vi "Process.vi"(8 "error in":errorcluster, 11 "Plugin in":refnum<class "Tone Measurements.lvclass">) -> (0 "error out":errorcluster, 3 "Plugin out":refnum<class "Tone Measurements.lvclass">)   [LabVIEW 2025, in "Tone Measurements.lvlib" / "Tone Measurements.lvclass"]
uses:
  Tone Measurements.lvclass
  C:/Program Files/National Instruments/LabVIEW 2025/vi.lib/FlexLogger/SDK/PluginSDK.lvlibp/PEFClasses/SDK/Plugin/Plugin.lvclass
  <vilib>/addons/_NISVFA/_Shared subVIs/Controls/svc_Window.ctl
  Tone Measurements.lvclass/Tone Measurements.ctl
  <vilib>/addons/_NISVFA/_Shared subVIs/Data Objects/Data/Data.lvclass/Data.ctl
  <vilib>/addons/_NISVFA/_Shared subVIs/Data Objects/Data/Read Data Increment.vi
  <vilib>/addons/_NISVFA/_Shared subVIs/Data Objects/Data/Read Data Attributes.vi
  <vilib>/addons/_NISVFA/_Shared subVIs/Data Objects/subVIs/Get Data Sample Interval (dt).vi
  <vilib>/addons/_NISVFA/_Shared subVIs/Common/sv_Get NI Property Name String.vi
  <vilib>/addons/_NISVFA/_Shared subVIs/Data Objects/Waveforms (DBL)/Waveforms (N Ch).lvclass
  C:/Program Files/NI/LVAddons/nisvt/1/vi.lib/addons/_NISVFA/_Shared subVIs/Data Objects/Data/Data.lvclass
  <vilib>/addons/_NISVFA/_Shared subVIs/Data Objects/Waveforms (DBL)/SV Read Newest Data.vi
  <vilib>/FlexLogger/SDK/PluginSDK.lvlibp/PEFClasses/SDK/Plugin/DataHelpers/Write 1D Wfm (DBL)_v2.vi
  C:/Program Files/National Instruments/LabVIEW 2025/vi.lib/FlexLogger/SDK/PluginSDK.lvlibp/PEFClasses/SDK/Processing Element/Processing Element.lvclass
  C:/dev/dsb/niflexlogger-plugins/PDK plugins/Tone Measurements/Tone Measurements.lvclass
  <vilib>/FlexLogger/SDK/PluginSDK.lvlibp/PEFClasses/SDK/Plugin/Plugin.lvclass
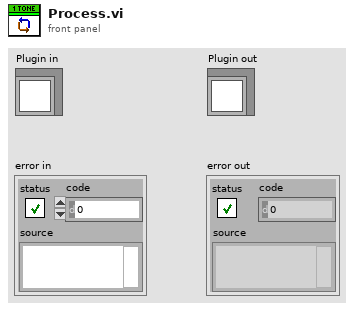
[diagram p1: front panel]
types:
  T1 = cluster{"start frequency":dbl, "stop frequency":dbl}
  T2 = typedef "svc_Window.ctl" = u32
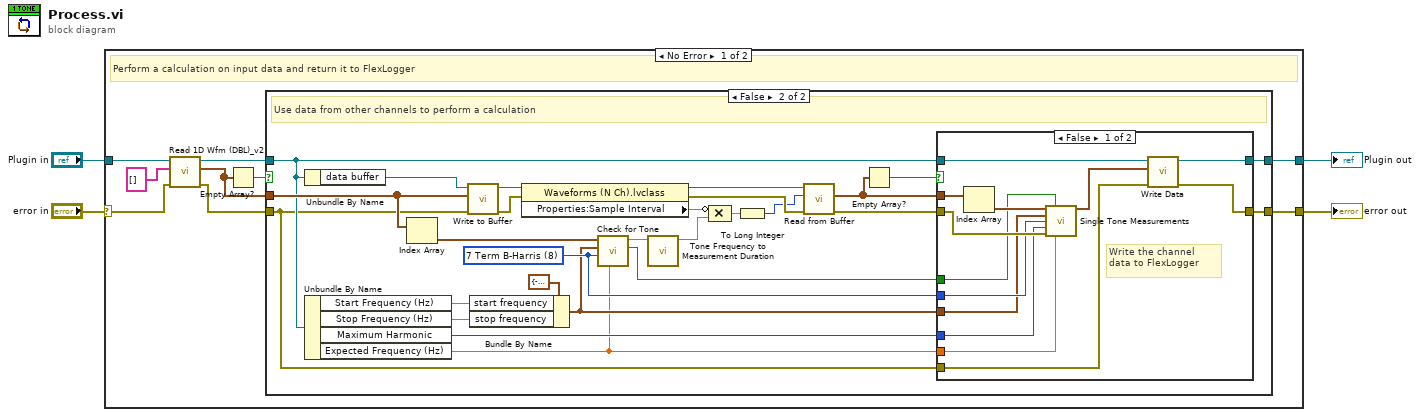
[diagram p0: block diagram]
diagram:
  n1 = case shown="No Error" "error in" {
    selector: "error in" -> [w12 w58]
    tunnel: [w10 w59] -> w1
    tunnel: "Plugin in" -> [w13 w59]
    tunnel: [w11 w58] -> w2
    frame No Error {
      # "Perform a calculation on input data and return it to FlexLogger"
      n2 = call <vilib>:"Read 1D Wfm (DBL)_v2.vi"("error in (no error)"=w12, "Unique Identifiers (empty = all)"=string[] [] ("Unique Channel Identifers (empty = all)"), "Plugin in"=w13) -> ("error out"=w5:errorcluster, "Data"=w6:waveform(dbl)[], "Plugin out"=w9:refnum<class "Tone Measurements.lvclass">)  [unwired: 5 in, 1 out]
      n3 = Empty Array?(array=w6) -> (empty?=w7:bool)
      n4 = case shown="False" w7 {
        tunnel: [w14 w42] -> w11
        tunnel: [w15 w41] -> w10
        tunnel: w9 -> [w15 w32]
        tunnel: w6 -> [_ w37]
        tunnel: w5 -> [w14 w18]
        frame True {
          # "No channels sending data to the plugin"
        }
        frame False {
          w31 = T2 8 items=["None"=0, "Hanning"=1, "Hamming"=2, "Blackman-Harris"=3, "Exact Blackman"=4, "Blackman"=5, "Flat Top"=6, "4 Term B-Harris "=7, "7 Term B-Harris"=8, "Low Sidelobe"=9, "Force"=64, "Exponential"=65, "Blackman Nuttall"=11, "Triangle"=30, "Bartlett-Hanning"=31, "Bohman"=32, "Parzen"=33, "Welch"=34, "Kaiser"=60, "Dolph-Chebyshev"=61, "Gaussian"=62] ("window")
          # "Use data from other channels to perform a calculation"
          n5 = Unbundle By Name(w32) -> ("data buffer"=w40:refnum<data-value>)
          n6 = Unbundle By Name(w32) -> ("Start Frequency (Hz)"=w35:dbl, "Stop Frequency (Hz)"=w36:dbl, "Maximum Harmonic"=w33:i32, "Expected Frequency (Hz)"=w28:dbl)
          n7 = Index Array(array=w37) -> (element=w29:waveform(dbl))  [unwired: 1 in]
          n8 = call <vilib>:"Write to Buffer.vi"("error in (no error)"=w18, "waveforms"=w37, "buffer"=w40) -> ("error out"=w24:errorcluster, "buffer out"=w26:refnum<data-value>)  [unwired: 6 in, 1 out]
          n9 = Bundle By Name(cluster=T1 {"start frequency"=-1.0, "stop frequency"=-1.0} ("frequency range"), "start frequency"=w35, "stop frequency"=w36) -> (w30:T1)
          n10 = property class="Waveforms (N Ch).lvclass"(reference=w26, error in=w24) -> (reference out=w25:refnum<data-value>, error out=w23:errorcluster, "Properties:Sample Interval"=w22:dbl)
          n11 = call "Check for Tone.vi"("expected frequency (Hz)"=w28, "window"=w31, "frequency range"=w30, "waveform"=w29) -> ("tone detected?"=w16:bool, "frequency"=w27:dbl)  [unwired: 5 in, 1 out]
          n12 = call "Tone Frequency to Measurement Duration.vi"("tone frequency"=w27) -> ("measurement duration"=w21:dbl)  [unwired: 10 in]
          n13 = Compound Arithmetic op=MULTIPLY(invert w22, w21) -> (w20:dbl)
          n14 = To Long Integer(number=w20) -> (32bit integer=w19:i32)
          n15 = call-poly <vilib>:"Read from Buffer.vi"("error in (no error)"=w23, "block length (-1 = all)"=w19, "buffer"=w25) -> ("error out"=w38:errorcluster, "waveforms subset"=w39:waveform(dbl)[])  [unwired: 5 in, 2 out]
          n16 = Empty Array?(array=w39) -> (empty?=w17:bool)
          n17 = case shown="False" w17 {
            tunnel: [w55 w56] -> w42
            tunnel: [w54 w57] -> w41
            tunnel: w32 -> [w52 w57]
            tunnel: w39 -> [w51 _]
            tunnel: w38 -> [w49 _]
            tunnel: w33 -> [w48 _]
            tunnel: w30 -> [w45 _]
            tunnel: w31 -> [w46 _]
            tunnel: w28 -> [w47 _]
            tunnel: w18 -> [w43 w56]
            tunnel: w16 -> [w44 _]
            frame False {
              # "Write the channel data to FlexLogger"
              n18 = Index Array(array=w51) -> (element=w50:waveform(dbl))  [unwired: 1 in]
              n19 = call "Single Tone Measurements.vi"("scaled signals [EU]"=w50, "tone detected"=w44, "frequency range"=w45, "window"=w46, "Maximum Harmonic"=w48, "error in"=w49, "Expected Frequency (Hz)"=w47) -> ("single-tone measurements"=w53:waveform(dbl)[])  [unwired: 7 in, 1 out]
              n20 = call-poly <vilib>:"Write Data.vi"("error in (no error)"=w43, "Data"=w53, "Plugin in"=w52) -> ("error out"=w55:errorcluster, "Plugin out"=w54:refnum<class "Tone Measurements.lvclass">)  [unwired: 7 in]
            }
            frame True {
            }
          }
        }
      }
    }
    frame Error {
    }
  }
  "error out" <- w2
  "Plugin out" <- w1
